vi "Read Attributes.vi"(11 "Send Update Status Msg":refnum<class "Send Update Status Msg.lvclass">) -> (2 "Payload":cluster{"System_Status":T1})   [LabVIEW 2019, in "Send Update Status Msg.lvclass"]
uses:
  Send Update Status Msg.lvclass
  builds/Engine/Engine.lvlibp/Custom Controls/System Status.ctl
  Send Update Status Msg.lvclass/Send Update Status Msg.ctl
  builds/Engine/Engine.lvlibp/Project/Engine.lvclass
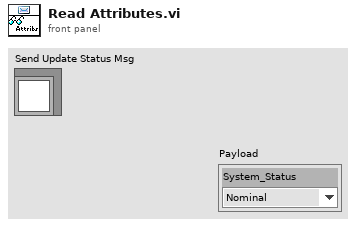
[diagram p1: front panel]
types:
  T1 = typedef "Engine.lvlibp/Engine.lvclass/System Status.ctl" = enum16{"Nominal", "Error", "Warning"}
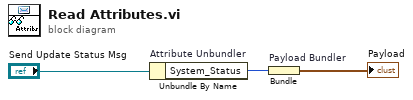
[diagram p0: block diagram]
diagram:
  n1 = Unbundle By Name "Attribute Unbundler"("Send Update Status Msg") -> ("System_Status"=w1:T1)
  n2 = Bundle "Payload Bundler"("System_Status"=w1) -> (→"Payload":cluster{"System_Status":T1})  [unwired: 1 in]
